vi "Translate.vi"(10 "Message In":refnum<class "MSG.lvclass">, 11 "Translator in":refnum<class "AddOuterEnvelope.lvclass">) -> (2 "Translated Message":refnum<class "MSG.lvclass">, 3 "Translator out":refnum<class "AddOuterEnvelope.lvclass">)   [LabVIEW 2011, in "Messenging.lvlib" / "AddOuterEnvelope.lvclass"]
uses:
  AddOuterEnvelope.lvclass
  TextVarientMessage/MSG.lvclass
  AddOuterEnvelope.lvclass/AddOuterEnvelope.ctl
  TextVarientMessage/Write VarMessage.vi
  VarMessage/VarMessage.lvclass
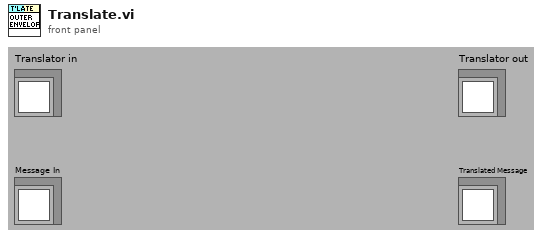
[diagram p1: front panel]
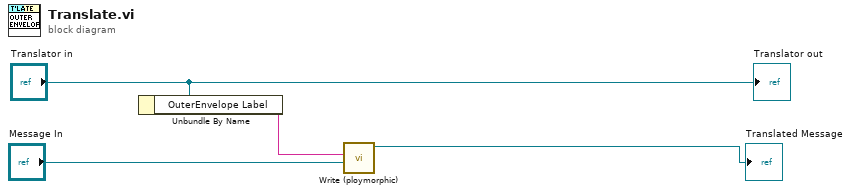
[diagram p0: block diagram]
diagram:
  n1 = Unbundle By Name("Translator in") -> ("OuterEnvelope Label"=w2:string)
  n2 = call-poly "Write (ploymorphic).vi"("Varient"="Message In", "Label"=w2) -> ("Message"=→"Translated Message":refnum<class "VarMessage.lvclass">)  [unwired: 1 in, 8 out]
  "Translator out" <- "Translator in"
